vi "WFGConfigureCarrierSingleCh.vi"(0 "object in":refnum<class "AD2_WFG_SDK.lvclass">, 2 "Ch":T1={"idxChannel"=0, "Settings out of range"=FALSE, "Carrier"={"Frequency (Hz)"=1000.0, "Amplitude (V)"=1.0, "Offset(V)"=0.0, "Symmetry(%) "=50.0, "Phase(Deg)"=0.0, "Function"=1, "Enable"=FALSE}, "Trigger"={"secRun(0=Cont)"=0.0, "secWait"=0.0, "cRepeat(0=inf)"=0, "Repeat Trigger"=FALSE, "TrigrSrc"=enum."trigrsrcNone"}, "FM Mod"={"Frequency (Hz)"=1000.0, "Amplitude (%)"=1.0, "Offset(V)"=0.0, "Symmetry(%) "=50.0, "Phase(Deg)"=0.0, "Function 2"=1, "Enable"=FALSE}} {"FM Mod"."Function 2" items=["DC"=0, "Sine"=1, "Square"=2, "Triangle"=3, "RampUp"=4, "RampDown"=5, "Noise"=6, "Pulse"=7, "Custom"=30]; "Carrier"."Function" items=["DC"=0, "Sine"=1, "Square"=2, "Triangle"=3, "RampUp"=4, "RampDown"=5, "Noise"=6, "Pulse"=7, "Custom"=30]}, 5 "error in (no error)":errorcluster) -> (14 "object out":refnum<class "AD2_WFG_SDK.lvclass">, 19 "error out":errorcluster)   [LabVIEW 2019, in "AD2_WFG_SDK.lvclass"]
uses:
  AD2_WFG_SDK.lvclass
  WFGCh.ctl
  AD2TriggerSources.ctl
  Olasdwf/Olasdwf.lvlib
  AD2_SDK_class/AD2_SDK.lvclass
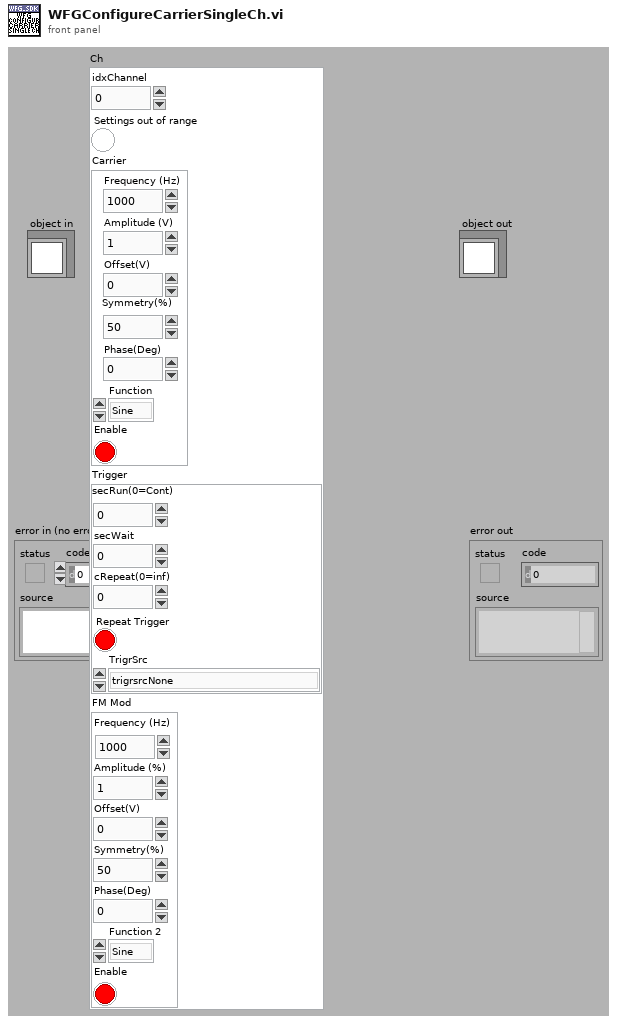
[diagram p1: front panel]
types:
  T1 = typedef "AD2_WFG_SDK.lvclass/WFGCh.ctl" = cluster{"idxChannel":i32, "Settings out of range":bool, "Carrier":cluster{"Frequency (Hz)":dbl, "Amplitude (V)":dbl, "Offset(V)":dbl, "Symmetry(%) ":dbl, "Phase(Deg)":dbl, "Function":u16, "Enable":bool}, "Trigger":cluster{"secRun(0=Cont)":dbl, "secWait":dbl, "cRepeat(0=inf)":i32, "Repeat Trigger":bool, "TrigrSrc":T2}, "FM Mod":cluster{"Frequency (Hz)":dbl, "Amplitude (%)":dbl, "Offset(V)":dbl, "Symmetry(%) ":dbl, "Phase(Deg)":dbl, "Function 2":u16, "Enable":bool}}
  T2 = typedef "AD2_SDK.lvclass/AD2TriggerSources.ctl" = enum8{"trigrsrcNone", "trigsrcPC", "trigsrcDetectorAnalogIn", "trigsrcDetectorDigitalIn", "trigsrcAnalogIn", "trigsrcDigitalIn", "trigsrcDigitalOut", "trigsrcAnalogOut1", "trigsrcAnalogOut2", "trigsrcAnalogOut3", "trigsrcAnalogOut4", "trigsrcExternal1", "trigsrcExternal2", "trigsrcExternal3", "trigsrcExternal4", ""}
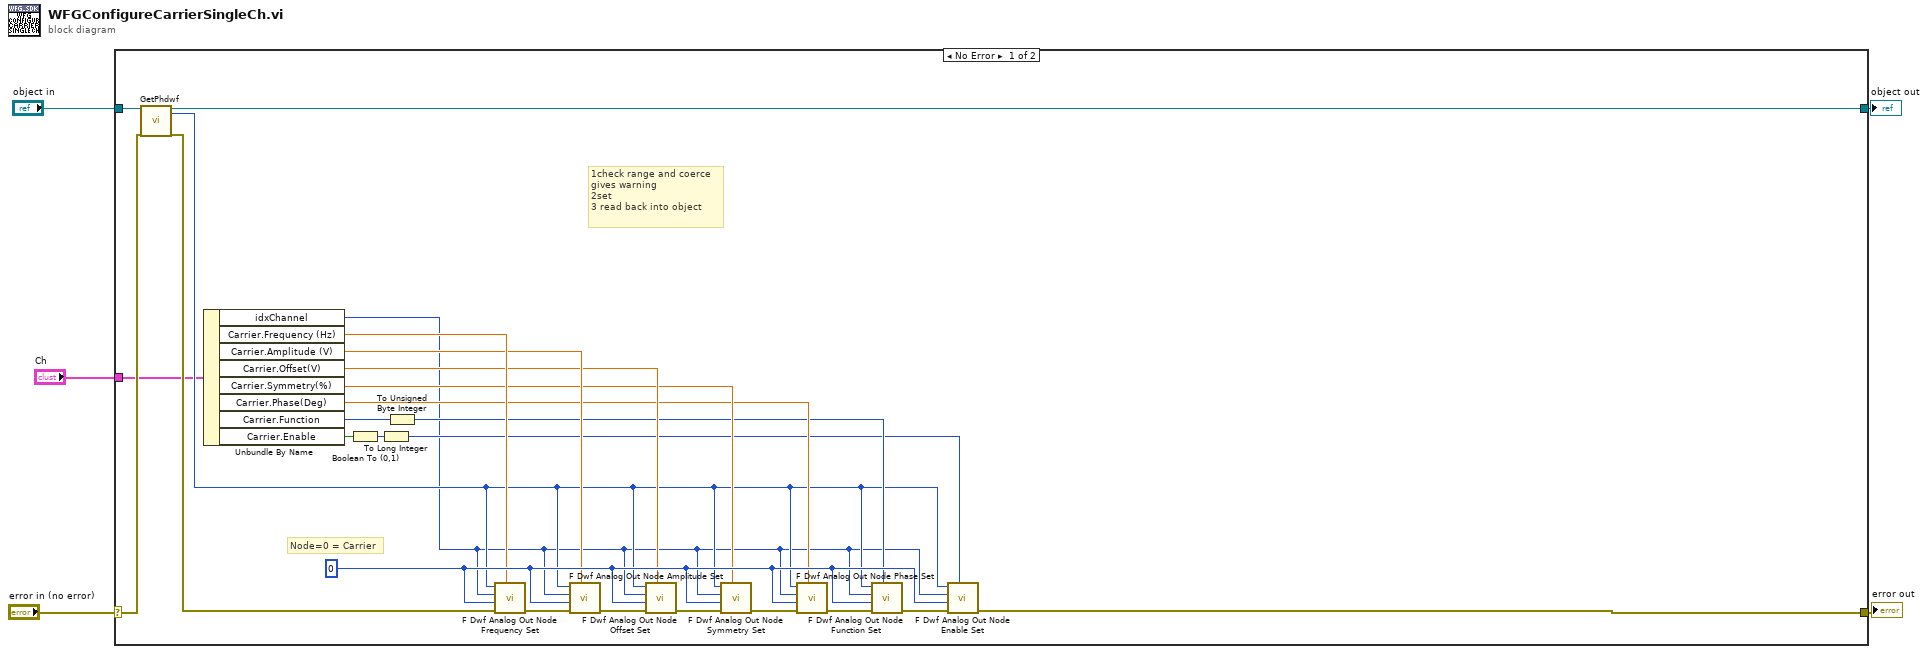
[diagram p0: block diagram]
diagram:
  n1 = case shown="No Error" "error in (no error)" {
    selector: "error in (no error)" -> [w25 w32]
    tunnel: [w6 w32] -> w4
    tunnel: [w27 w31] -> w2
    tunnel: "object in" -> [w26 w31]
    tunnel: "Ch" -> [w7 _]
    frame No Error {
      w18 = 0 ("node")
      # "1check range and coerce\ngives warning\n2set\n3 read back into object"
      # "Node=0 = Carrier"
      n2 = call-dynamic "GetPhdwf.vi"("object in"=w26, "error in (no error)"=w25) -> ("object out"=w27:refnum<class "AD2_WFG_SDK.lvclass">, "phdwf"=w9:i32, "error out"=w10:errorcluster)  [unwired: 15 in]
      n3 = Unbundle By Name(w7) -> ("idxChannel"=w8:i32, "Carrier.Frequency (Hz)"=w17:dbl, "Carrier.Amplitude (V)"=w16:dbl, "Carrier.Offset(V)"=w15:dbl, "Carrier.Symmetry(%)"=w14:dbl, "Carrier.Phase(Deg)"=w13:dbl, "Carrier.Function"=w29:u16, "Carrier.Enable"=w28:bool)
      n4 = Boolean To (0,1)(Boolean=w28) -> (0, 1=w30:i16)
      n5 = To Long Integer(number=w30) -> (32bit integer=w11:i32)
      n6 = To Unsigned Byte Integer(number=w29) -> (unsigned 8bit integer=w12:u8)
      n7 = call "F Dwf Analog Out Node Frequency Set.vi"("hzFrequency"=w17, "error in (no error)"=w10, "node"=w18, "idxChannel"=w8, "hdwf"=w9) -> ("error out"=w20:errorcluster)  [unwired: 5 in, 1 out]
      n8 = call "F Dwf Analog Out Node Amplitude Set.vi"("vAmplitude"=w16, "error in (no error)"=w20, "node"=w18, "idxChannel"=w8, "hdwf"=w9) -> ("error out"=w21:errorcluster)  [unwired: 5 in, 1 out]
      n9 = call "F Dwf Analog Out Node Offset Set.vi"("vOffset"=w15, "error in (no error)"=w21, "node"=w18, "idxChannel"=w8, "hdwf"=w9) -> ("error out"=w22:errorcluster)  [unwired: 5 in, 1 out]
      n10 = call "F Dwf Analog Out Node Symmetry Set.vi"("percentageSymmetry"=w14, "error in (no error)"=w22, "node"=w18, "idxChannel"=w8, "hdwf"=w9) -> ("error out"=w23:errorcluster)  [unwired: 5 in, 1 out]
      n11 = call "F Dwf Analog Out Node Phase Set.vi"("degreePhase"=w13, "error in (no error)"=w23, "node"=w18, "idxChannel"=w8, "hdwf"=w9) -> ("error out"=w24:errorcluster)  [unwired: 5 in, 1 out]
      n12 = call "F Dwf Analog Out Node Function Set.vi"("func"=w12, "error in (no error)"=w24, "node"=w18, "idxChannel"=w8, "hdwf"=w9) -> ("error out"=w19:errorcluster)  [unwired: 5 in, 1 out]
      n13 = call "F Dwf Analog Out Node Enable Set.vi"("fEnable"=w11, "error in (no error)"=w19, "node"=w18, "idxChannel"=w8, "hdwf"=w9) -> ("error out"=w6:errorcluster)  [unwired: 5 in, 1 out]
    }
    frame Error {
    }
  }
  "error out" <- w4
  "object out" <- w2
